vi "applyDelays.vi"(8 "error in (no error)":errorcluster, 11 "ScriptEventList in":refnum<class "ScriptEventList.lvclass">) -> (0 "error out":errorcluster, 3 "ScriptEventList out":refnum<class "ScriptEventList.lvclass">)   [LabVIEW 2009, in "Tools.lvlib" / "Scripting.lvlib" / "ScriptEventList.lvclass"]
uses:
  ScriptEventList.lvclass
  ScriptEventList.lvclass/ScriptEventList.ctl
  ScriptEvent.lvclass
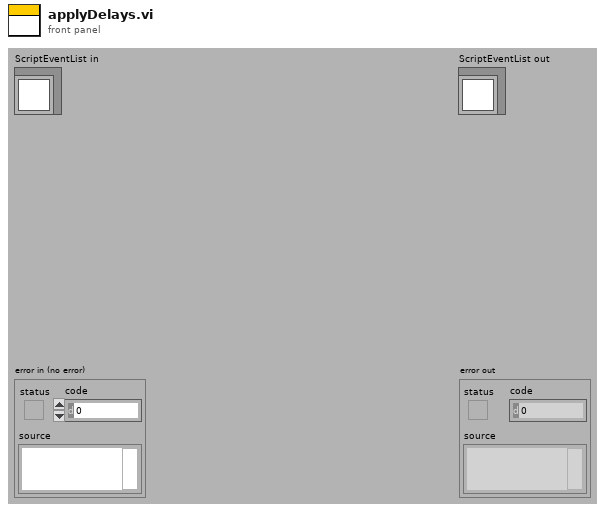
[diagram p1: front panel]
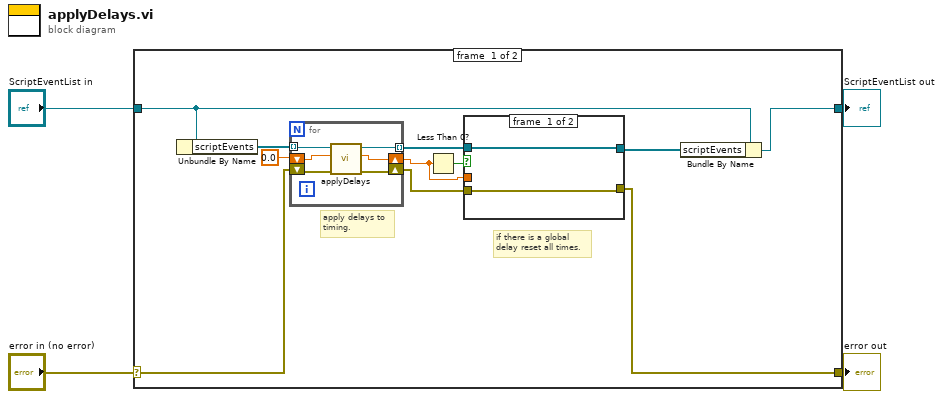
[diagram p0: block diagram]
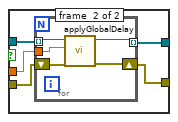
[diagram p2: hidden frame]
diagram:
  n1 = case shown="No Error" "error in (no error)" {
    selector: "error in (no error)" -> [w13 w35]
    tunnel: [w8 w35] -> w3
    tunnel: [w5 w34] -> w1
    tunnel: "ScriptEventList in" -> [w6 w34]
    frame #0 {
      # "if there is a global\ndelay reset all times."
      # "apply delays to\ntiming."
      n2 = Unbundle By Name(w6) -> ("scriptEvents"=w15:refnum<class "ScriptEvent.lvclass">[])
      n3 = for {
        tunnel: w15 -> [w33] mode=indexing
        shift-right: [w31] -> w10
        shift-left: 0.0 -> [w32]
        shift-right: [w29] -> w9
        shift-left: w13 -> [w30]
        tunnel: [w28] -> w12 mode=indexing
        n4 = call "applyDelays.vi"("error in (no error)"=w30, "globalDelay"=w32, "ScriptEvent in"=w33) -> ("error out"=w29:errorcluster, "globalDelay out"=w31:dbl, "ScriptEvent out"=w28:refnum<class "ScriptEvent.lvclass">)  [unwired: 6 in]
      }
      n5 = Less Than 0?(x=w10) -> (x < 0?=w11:bool)
      n6 = case shown="True" w11 {
        tunnel: w12 -> [w17 w22]
        tunnel: w10 -> [_ w21]
        tunnel: w9 -> [w16 w20]
        tunnel: [w16 w19] -> w8
        tunnel: [w17 w18] -> w7
        frame #0 {
        }
        frame #1 {
          n7 = for {
            tunnel: w22 -> [w27] mode=indexing
            shift-right: [w24] -> w19
            shift-left: w20 -> [w25]
            tunnel: [w23] -> w18 mode=indexing
            tunnel: w21 -> [w26]
            n8 = call "applyGlobalDelay.vi"("error in (no error)"=w25, "globalDelay"=w26, "ScriptEvent in"=w27) -> ("error out"=w24:errorcluster, "ScriptEvent out"=w23:refnum<class "ScriptEvent.lvclass">)  [unwired: 7 in]
          }
        }
      }
      n9 = Bundle By Name(cluster=w6, "scriptEvents"=w7) -> (w5:refnum<class "ScriptEventList.lvclass">)
    }
    frame #1 {
    }
  }
  "error out" <- w3
  "ScriptEventList out" <- w1
